vi "Process File.vi"(8 "error in (no error)":errorcluster, 10 "Result in":refnum<class "Acquired Result.lvclass">, 11 "Resampler in":refnum<class "Resampler.lvclass">) -> (0 "error out":errorcluster, 2 "Result out":refnum<class "Acquired Result.lvclass">, 3 "Resampler out":refnum<class "Resampler.lvclass">)   [LabVIEW 2024, in "Resampler.lvclass"]
uses:
  Resampler.lvclass
  Resampler.lvclass/Resampler.ctl
  NHMFL_Core/Libraries/Instruments/Results/Acquired Result/Acquired Result.lvclass
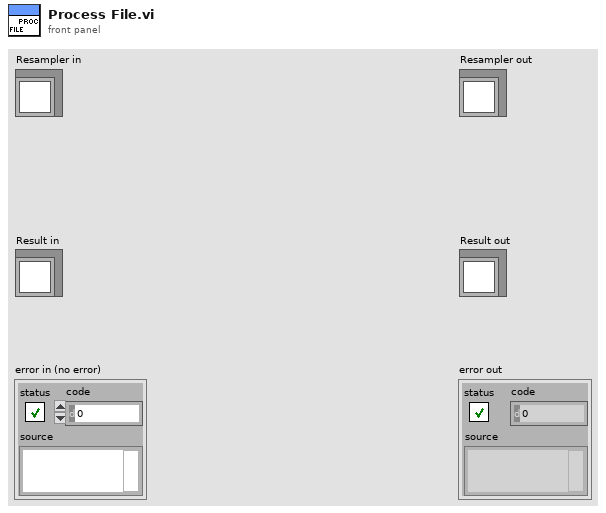
[diagram p1: front panel]
types:
  T1 = enum16{"open", "open or create", "create or replace", "create", "open (read-only)"}
  T2 = typedef "Resampler Configuration.ctl" = cluster{"Group":string, "Reference channel":string, "Channels to resample":string[]}
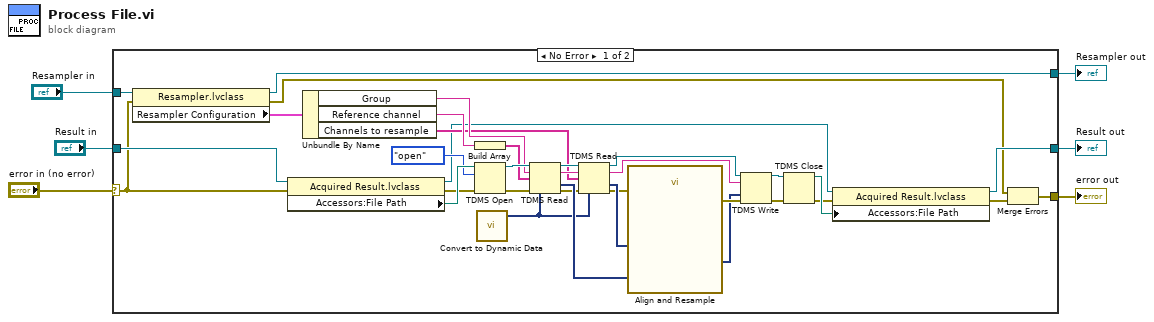
[diagram p0: block diagram]
diagram:
  n1 = case shown="No Error" "error in (no error)" {
    selector: "error in (no error)" -> [w38 w42]
    tunnel: "Result in" -> [w40 w43]
    tunnel: "Resampler in" -> [w39 w41]
    tunnel: [w9 w42] -> w3
    tunnel: [w13 w43] -> w2
    tunnel: [w10 w41] -> w1
    frame No Error {
      n2 = property class="Resampler.lvclass"(reference=w39, error in=w38) -> (reference out=w10:refnum<class "Resampler.lvclass">, error out=w8:errorcluster, "Resampler Configuration"=w33:T2)
      n3 = property class="Acquired Result.lvclass"(reference=w40, error in=w38) -> (reference out=w7:refnum<class "Acquired Result.lvclass">, error out=w20:errorcluster, "Accessors:File Path"=w35:path)
      n4 = Unbundle By Name(w33) -> ("Group"=w32:string, "Reference channel"=w31:string, "Channels to resample"=w26:string[])
      n5 = Build Array(w31) -> (w30:string[])
      n6 = TDMS Open(8:w20, 10:T1."open" ("operation (0:open)"), 11:w35) -> (0:w37:errorcluster, 3:w36:refnum<k34>)  [unwired: 4 in]
      n7 = call "Convert to Dynamic Data"() -> ("Dynamic Data Type"=w24:dynamicdata)  [unwired: 4 in]
      n8 = TDMS Read(0:w36, 5:w32, 7:w30, 11:w37, 12:w24) -> (4:w28:refnum<k34>, 6:w27:string, 10:w29:dynamicdata, 15:w21:errorcluster)  [unwired: 3 in, 2 out]
      n9 = TDMS Read(0:w28, 5:w27, 7:w26, 11:w21, 12:w24) -> (4:w23:refnum<k34>, 6:w18:string, 10:w25:dynamicdata, 15:w22:errorcluster)  [unwired: 3 in, 2 out]
      n10 = call "Align and Resample"("Reference Signal"=w29, "error in (no error)"=w22, "Signals"=w25) -> ("error out"=w19:errorcluster, "Resampled Signals"=w17:dynamicdata)  [unwired: 6 in, 1 out]
      n11 = TDMS Write(0:w23, 5:w18, 9:w17, 11:w19) -> (4:w15:refnum<k34>, 15:w16:errorcluster)  [unwired: 2 in, 2 out]
      n12 = TDMS Close(8:w16, 11:w15) -> (0:w12:errorcluster, 3:w14:path)
      n13 = property class="Acquired Result.lvclass"(reference=w7, error in=w12, "Accessors:File Path"=w14) -> (reference out=w13:refnum<class "Acquired Result.lvclass">, error out=w11:errorcluster)
      n14 = Merge Errors(w8, w11) -> (w9:errorcluster)
    }
    frame Error {
    }
  }
  "error out" <- w3
  "Resampler out" <- w1
  "Result out" <- w2
